vi "TestFitter.vi"() -> ()   [LabVIEW 2014, in "AnalysisPlugins.lvlib" / "PmuAnalysis.lvclass"]
uses:
  PmuAnalysis.lvclass
  AnalysisPluginBaseClass/Typedefs/clAnalysisConfig.ctl
  Typedefs/PmuData.ctl
  AnalysisPluginBaseClass/AnalysisPluginsBase.lvclass/AnalysisPluginsBase.ctl
  PmuAnalysis.lvclass/PmuAnalysis.ctl
  AnalysisPluginBaseClass/Accessors/Write Window.vi
  AnalysisPluginBaseClass/Accessors/Write SignalParams.vi
  AnalysisPluginBaseClass/Accessors/Write clConfig.vi
  AnalysisPluginBaseClass/Accessors/Write TestType.vi
  Accessors/Read PmuReport.vi
  AnalysisPluginBaseClass/AnalysisPluginsBase.lvclass
panel:
  out "error out":errorcluster
  out "PmuReport":T1 {"Synx" format="%#_4g"; "Timestamp" format="%.6f"}
  in  "Window":T2={"Timestamp"=3591878842.4333334, "Samples"=array6x1600[9600 elements], "Window Valid"=TRUE} {"Timestamp" format="%.6f"}
  in  "clConfig":T3={"F0"=60, "SettlingTime"=7.0, "AnalysisCycles"=20.0, "SampleRate"=4800.0, "NumChannels"=6, "TsOffset"=enum."start"}
  in  "SignalParams":dbl[](array[numeric])=[60.1, 0.0, 0.0, 0.0, 0.0, 0.0, 0.0, 0.0, 100.0, 100.0]
  # "Steady State Signals at 60.1 Hz"
  # "Fundamental Frequency"
  # "Harmonic Frequency"
  # "Interharmonic Frequency"
  # "Fundamental Initial Phase"
  # "Harmonic Initial Phase"
  # "Interharmonic Initial Phase"
  # "Harmonic Index"
  # "Interharmonic Index"
  # "Voltage Magnitude Index"
  # "Current Magnitude Index"
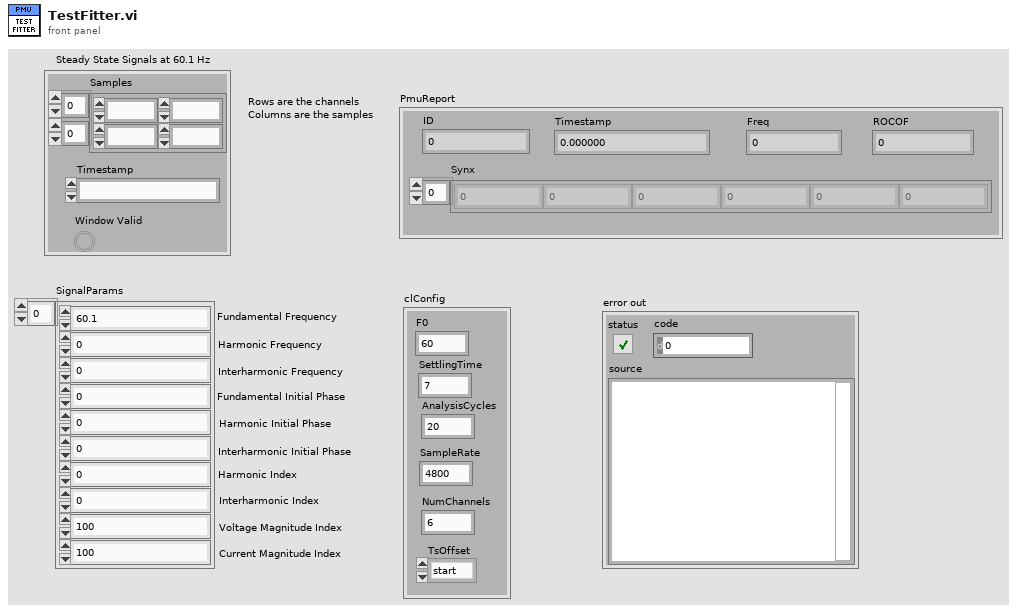
[diagram p1: front panel]
types:
  T1 = typedef "AnalysisPlugins.lvlib/PmuAnalysis.lvclass/PmuData.ctl" = cluster{"Timestamp":dbl, "Synx":cdb[], "Freq":dbl, "ROCOF":dbl, "ID":i16}
  T2 = cluster{"Timestamp":ext, "Samples":dbl[][], "Window Valid":bool}
  T3 = typedef "AnalysisPlugins.lvlib/AnalysisPluginsBase.lvclass/clAnalysisConfig.ctl" = cluster{"F0":u32, "SettlingTime":dbl, "AnalysisCycles":dbl, "SampleRate":dbl, "NumChannels":u32, "TsOffset":enum16{"start", "middle", "end"}}
  T4 = typedef "SensorPlugins.lvlib/PmuBase.lvclass/PmuData.ctl" = cluster{"Timestamp":dbl, "Synx":cdb[], "Freq":dbl, "ROCOF":dbl, "ID":i16}
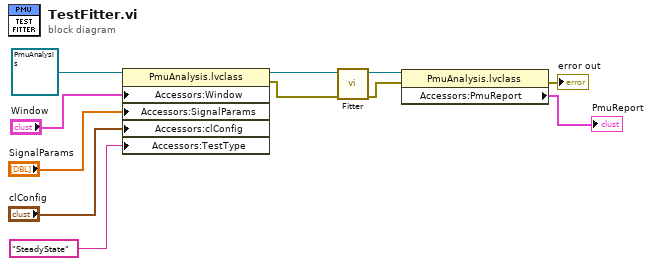
[diagram p0: block diagram]
diagram:
  n1 = property class="PmuAnalysis.lvclass"(reference=refnum<class "PmuAnalysis.lvclass"> refnum ("AnalysisPlugins.lvlib:PmuAnalysis.lvclass"), "Accessors:Window"="Window", "Accessors:SignalParams"="SignalParams", "Accessors:clConfig"="clConfig", "Accessors:TestType"="SteadyState") -> (reference out=w6:refnum<class "PmuAnalysis.lvclass">, error out=w5:errorcluster)  [unwired: 1 in]
  n2 = call-dynamic "Fitter.vi"("error in (no error)"=w5, "PmuAnalysis in"=w6) -> ("error out"=w2:errorcluster, "PmuAnalysis out"=w4:refnum<class "PmuAnalysis.lvclass">)  [unwired: 8 in]
  n3 = property class="PmuAnalysis.lvclass"(reference=w4, error in=w2) -> (error out=→"error out":errorcluster, "Accessors:PmuReport"=→"PmuReport":T4)  [unwired: 1 out]
